vi "Auto Drive.vi"(8 "heading":dbl, 9 "async":dbl, 10 "speed":dbl, 11 "y":dbl) -> (2 "isFinished?":bool)   [LabVIEW 2015]
uses:
  Common Code/Drivetrain Modes.ctl
  Robot Global Data.vi
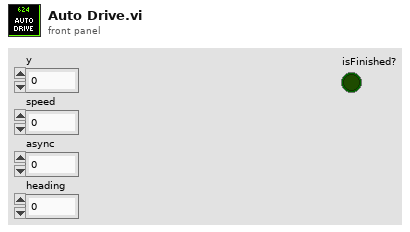
[diagram p1: front panel]
types:
  T1 = typedef "Drivetrain Modes.ctl" = enum16{"Climb", "Manual", "Ball Vision Targeting", "Goal Vision Targeting", "PID Distance Drive", "Hybrid"}
  T2 = typedef "Drivetrain Status Cluster.ctl" = cluster{"Modes":T1, "Y (Throttle)":dbl, "X (Steer)":dbl, "Gyro In Range?":bool, "Distance Drive Finished?":bool, "Stop Eject Lockout":bool, "Dist Drive Status":T3, "Y Target":dbl, "Heading Target":dbl, "Vision Target Aligned?":bool, "Gear":dbl, "1st Gear Time":dbl, "2nd Gear Time":dbl, "1st Gear Shifts":dbl, "2nd Gear Shifts":dbl}
  T3 = typedef "Dist Drive Status.ctl" = cluster{"Y In Range":bool, "X In Range":bool, "Gyro In Range":bool, "Y Dist":dbl, "X Dist":dbl, "Gyro":dbl}
  T4 = typedef "Drivetrain Commands.ctl" = cluster{"Y Power":dbl, "Turn Power":dbl, "1st Gear?":bool, "Modes":T1, "Heading Target":dbl, "X Max Speed":dbl, "Y Max Speed":dbl, "X Min Speed":dbl, "Y Min Speed":dbl, "Y Target":dbl, "Max Accel":dbl, "Max Velocity":dbl}
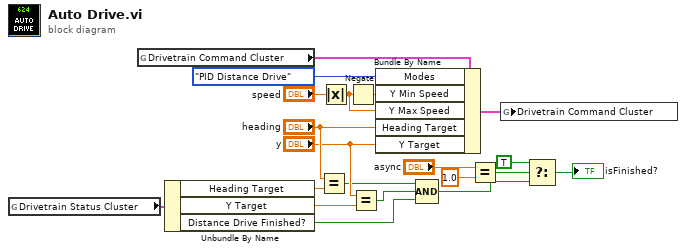
[diagram p0: block diagram]
diagram:
  n1 = global read "Robot Global Data.vi" "Drivetrain Status Cluster"() -> (w14:T2)
  n2 = global read "Robot Global Data.vi" "Drivetrain Command Cluster"() -> (w19:T4)
  n3 = Unbundle By Name(w14) -> ("Heading Target"=w13:dbl, "Y Target"=w11:dbl, "Distance Drive Finished?"=w7:bool)
  n4 = Equal?(x="heading", y=w13) -> (x = y?=w8:bool)
  n5 = Absolute Value(x="speed") -> (abs(x)=w15:dbl)
  n6 = Negate(x=w15) -> (-x=w16:dbl)
  n7 = Equal?(x="y", y=w11) -> (x = y?=w9:bool)
  n8 = Bundle By Name(cluster=w19, "Modes"=Drivetrain_Modes."PID Distance Drive", "Y Min Speed"=w16, "Y Max Speed"=w15, "Heading Target"="heading", "Y Target"="y") -> (w20:T4)
  n9 = Compound Arithmetic op=AND(w8, w9, w7) -> (w3:bool)
  n10 = Equal?(x="async", y=1.0) -> (x = y?=w4:bool)
  n11 = global write "Robot Global Data.vi" "Drivetrain Command Cluster"(w20) -> ()
  n12 = Select(t=TRUE, s=w4, f=w3) -> (s? t:f=→"isFinished?":bool)
